vi "MAC NSTART.vi"(0 "System no.":i32=1 min=1 max=4 step=1, 3 "Macro name":string, 4 "N":i32=1 min=0 max=20 step=1, 5 "error in":errorcluster, 6 "Arguments":string) -> (19 "error out":errorcluster)   [LabVIEW 2020]
doc: "Start macro N times. \n\nE-816: This command cannot be issued to a slave. Check controller manual to find out if MAC NSTART is supported. Arguments is not supported.\n\nC-887, F-206, M-8X0: Only for GCS syntax version = GCS 2.0 or higher (check with CSV?.vi. If CSV?.vi is not supported, syntax version is GCS 1.0). Use #8.vi to determine when macro execution has finished."
panel:
  # "Start macro N times."
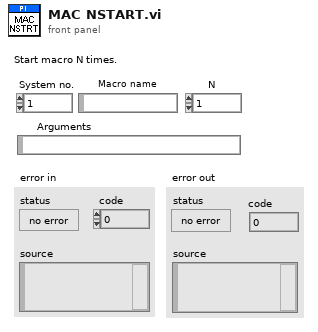
[diagram p1: front panel]
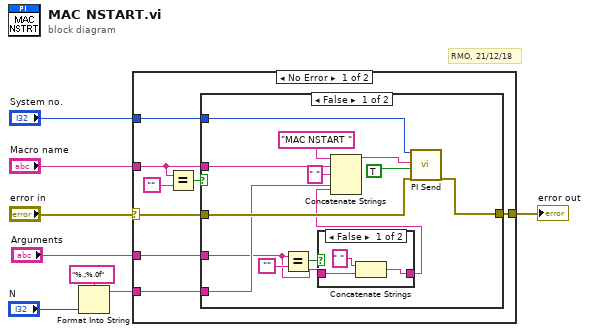
[diagram p0: block diagram]
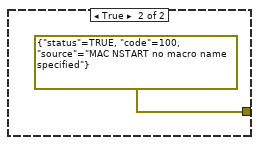
[diagram p3: hidden frame]
diagram:
  # "RMO, 21/12/18"
  n1 = Format Into String(format string="%.;%.0f" ("Format String"), "N") -> (resulting string=w3:string)  [unwired: 2 in, 1 out]
  n2 = case shown="No Error" "error in" {
    selector: "error in" -> [w9 w35]
    tunnel: "System no." -> [w16 _]
    tunnel: [w15 w35] -> w7
    tunnel: "Macro name" -> [w13 _]
    tunnel: w3 -> [w11 _]
    tunnel: "Arguments" -> [w10 _]
    frame No Error {
      n3 = Equal?(x=w13, y="") -> (x = y?=w12:bool)
      n4 = case shown="False" w12 {
        tunnel: w9 -> [w29 _]
        tunnel: w16 -> [w26 _]
        tunnel: [w24 errorcluster {"status"=TRUE, "code"=100, "source"="MAC NSTART no macro name specified"} ("error out")] -> w15
        tunnel: w13 -> [w23 _]
        tunnel: w11 -> [w22 _]
        tunnel: w10 -> [w17 _]
        frame False {
          n5 = Equal?(x=w17, y="") -> (x = y?=w19:bool)
          n6 = case shown="False" w19 {
            tunnel: w17 -> [w32 w33]
            tunnel: [w30 w33] -> w18
            frame False {
              n7 = Concatenate Strings(" ", w32) -> (w30:string)
            }
            frame True {
            }
          }
          n8 = Concatenate Strings("MAC NSTART ", w23, " " ("Substring"), w22, w18) -> (w25:string)
          n9 = call "PI Send.vi"("System no."=w26, "String to send"=w25, "Attach termination char.?"=TRUE ("Attach Linefeed?"), "error in"=w29) -> ("error out"=w24:errorcluster)  [unwired: 2 in, 13 out]
        }
        frame True {
        }
      }
    }
    frame Error {
    }
  }
  "error out" <- w7
